vi "Triangle_intersection.vi"(1 "No of Dynamic Facets":i32, 2 "No of Static Facets":i32, 3 "Body Bubble Rad":dbl, 4 "Body Centroid":dbl[](array[numeric]), 5 "Dynamic Facets":T1, 6 "Static Facets":T1) -> (0 "Collision?":bool)   [LabVIEW 2011]
uses:
  Facet_Array.ctl
  <vilib>/Analysis/baseanly.llb/Unit Vector (DBL).vi
  <vilib>/Analysis/baseanly.llb/Real Dot Product.vi
  <vilib>/Analysis/NI_AALBase.lvlib
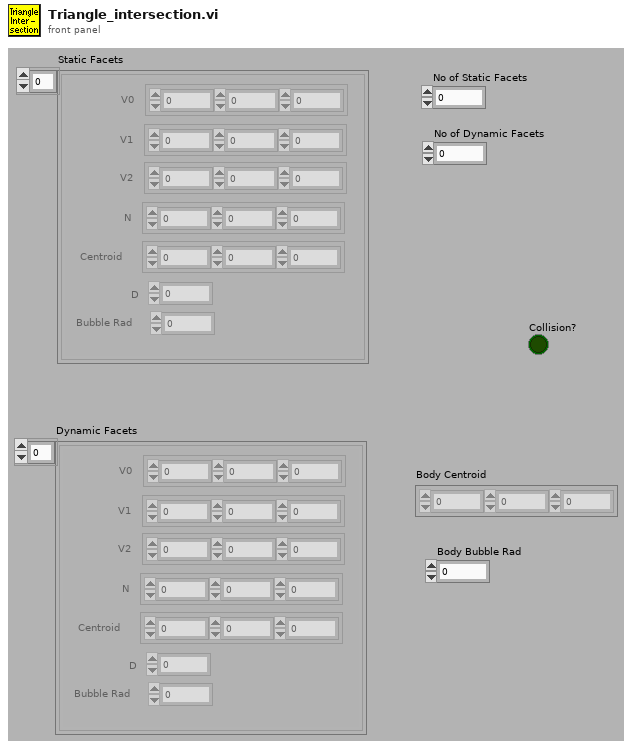
[diagram p1: front panel]
types:
  T1 = typedef "Facet_Array.ctl" = cluster{"V0":dbl[], "V1":dbl[], "V2":dbl[], "N":dbl[], "Centroid":dbl[], "D":dbl, "Bubble Rad":dbl}[]
  T2 = cluster{"V0":dbl[], "V1":dbl[], "V2":dbl[], "N":dbl[], "Centroid":dbl[], "D":dbl, "Bubble Rad":dbl}
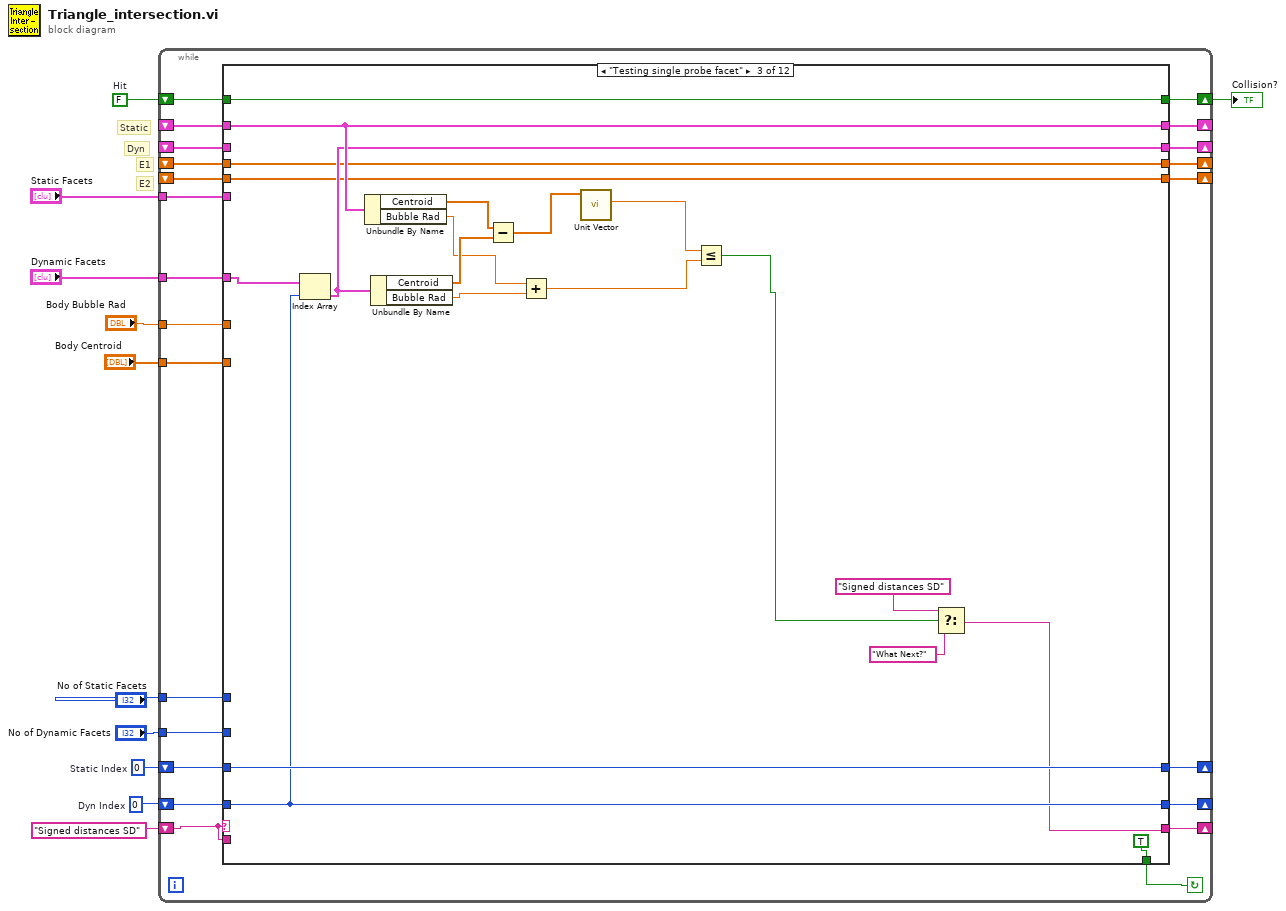
[diagram p0: block diagram]
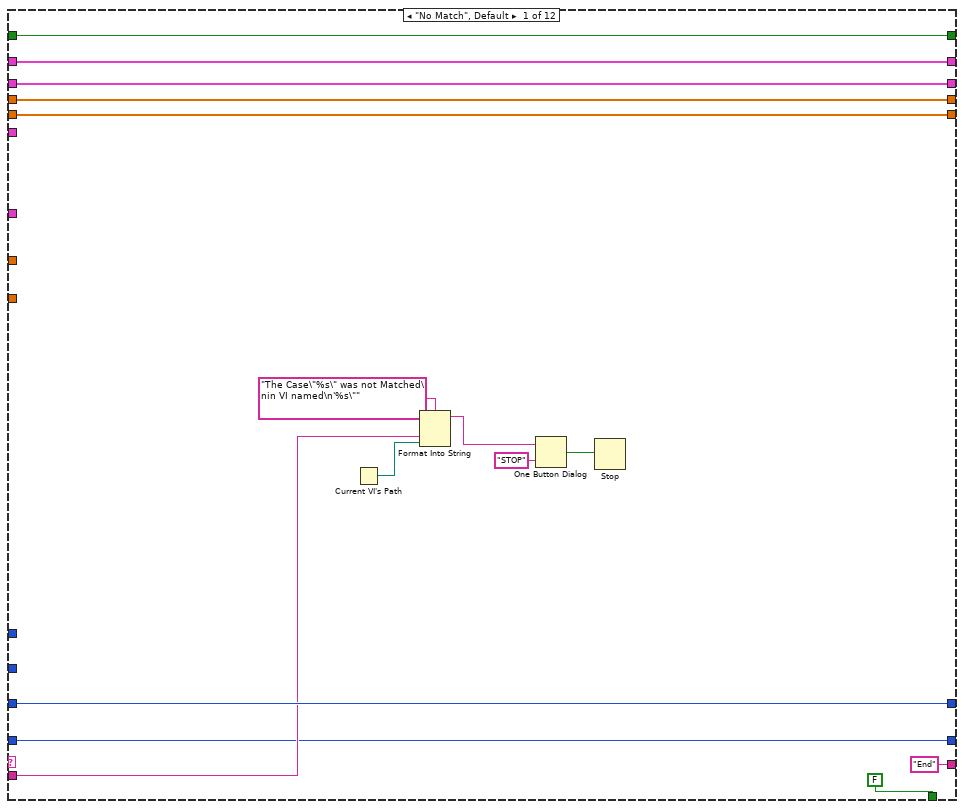
[diagram p2: hidden frame]
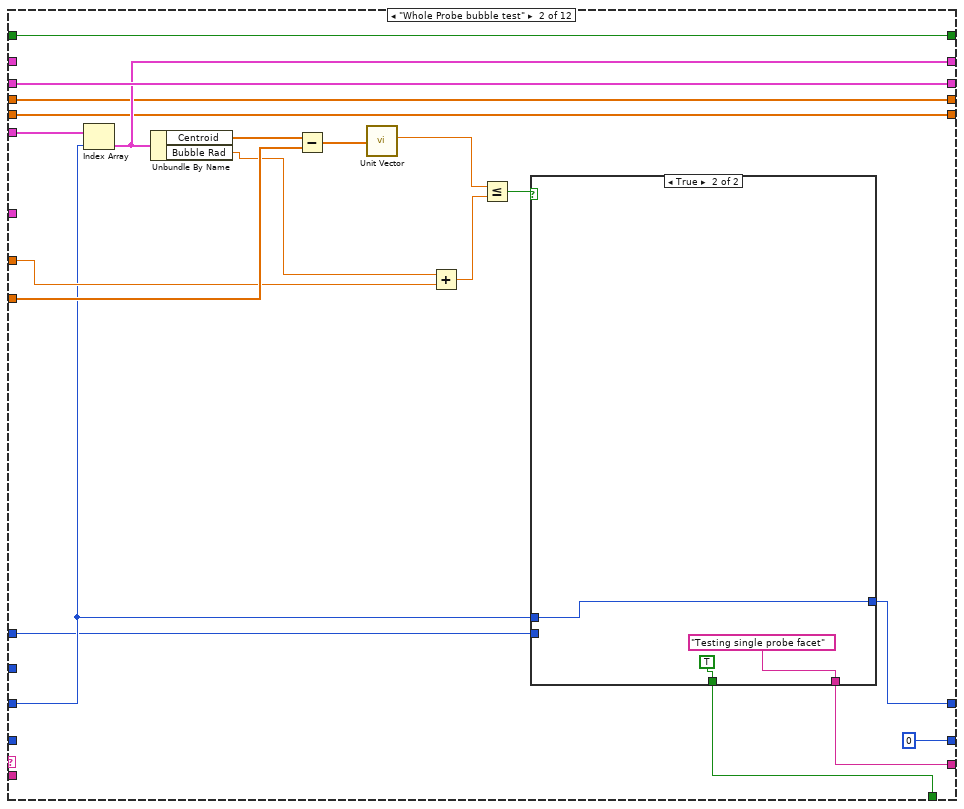
[diagram p3: hidden frame]
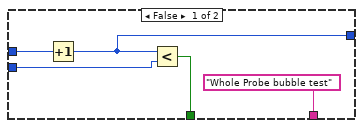
[diagram p4: hidden frame]
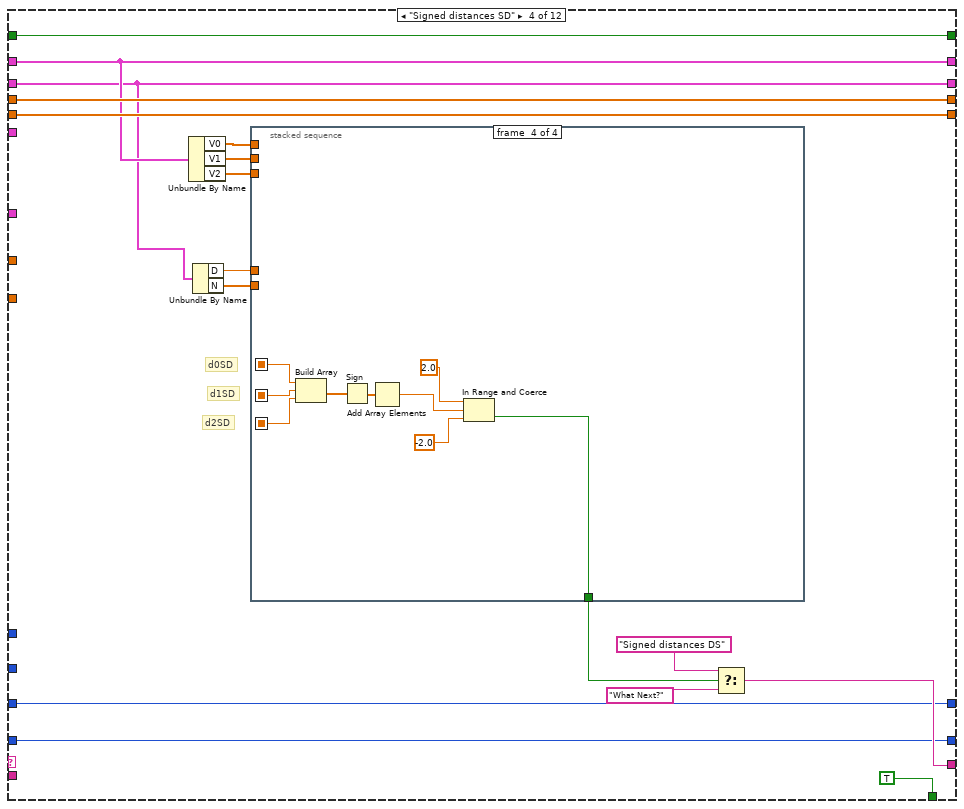
[diagram p5: hidden frame]
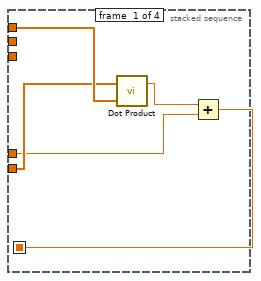
[diagram p6: hidden frame]
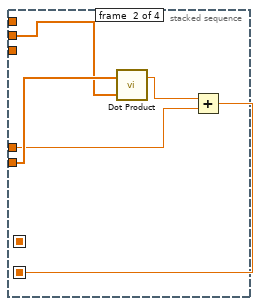
[diagram p7: hidden frame]
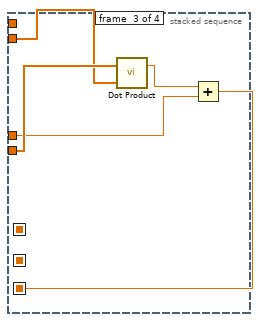
[diagram p8: hidden frame]
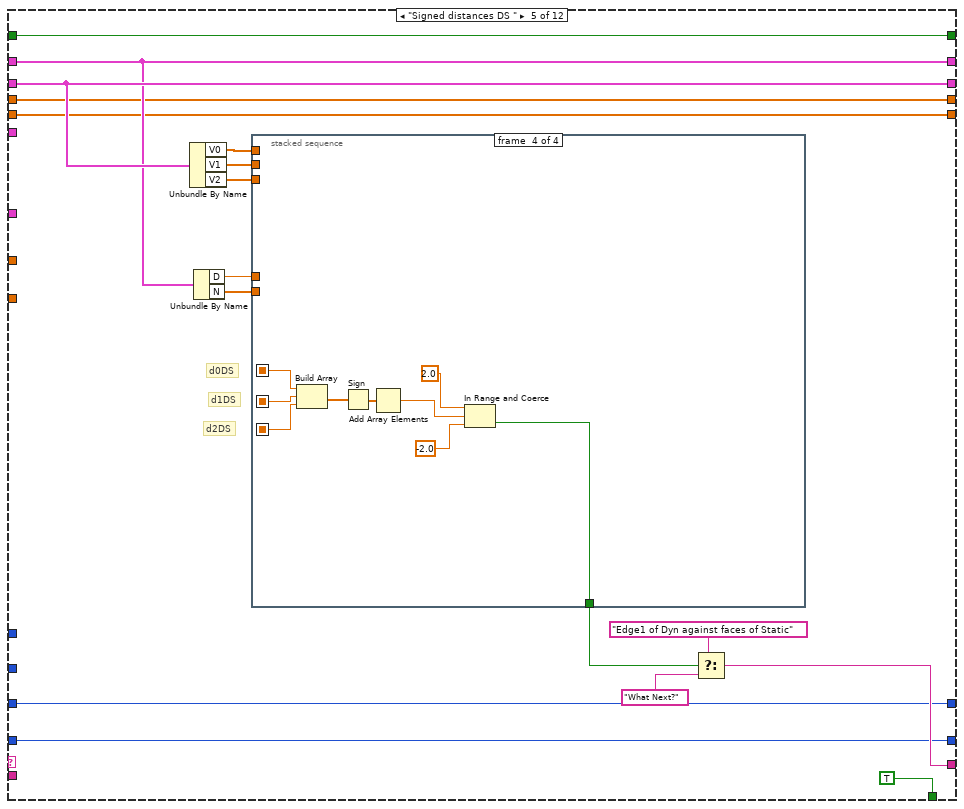
[diagram p9: hidden frame]
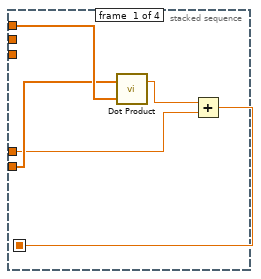
[diagram p10: hidden frame]
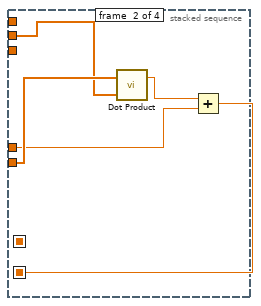
[diagram p11: hidden frame]
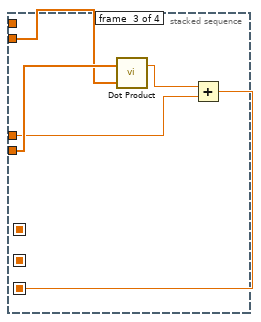
[diagram p12: hidden frame]
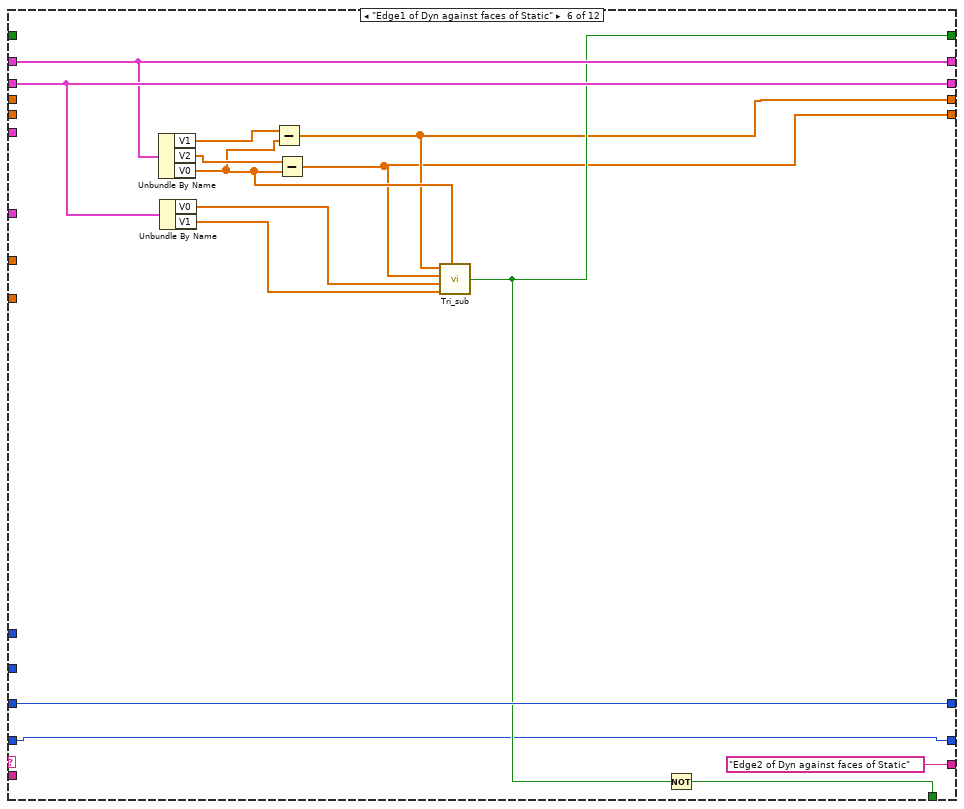
[diagram p13: hidden frame]
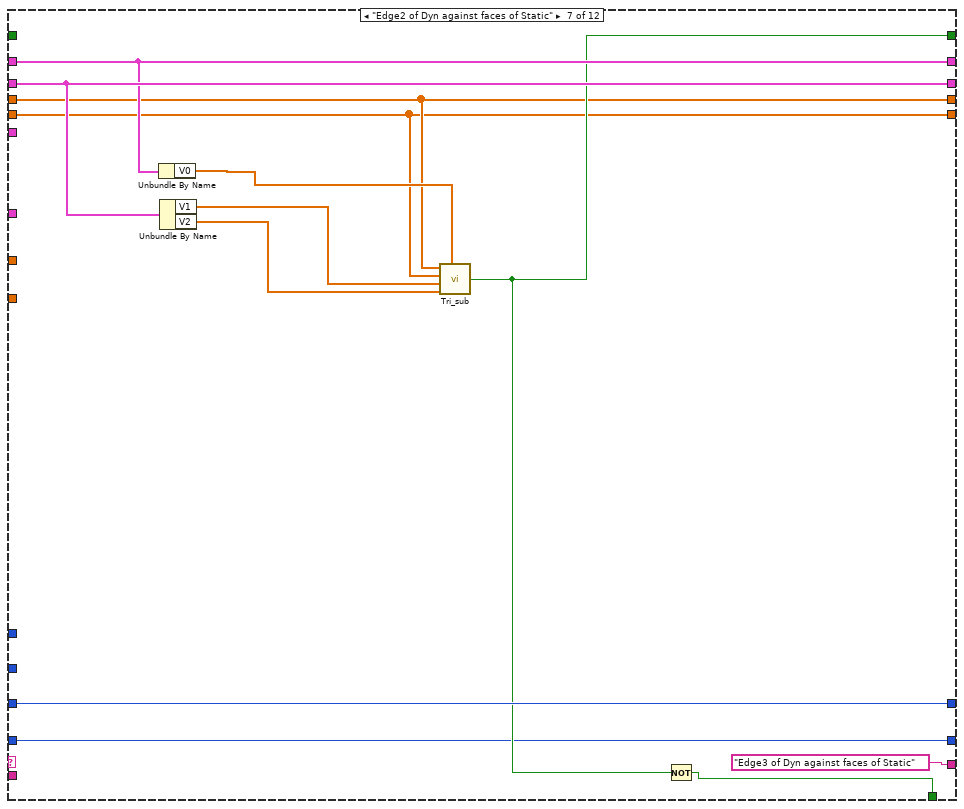
[diagram p14: hidden frame]
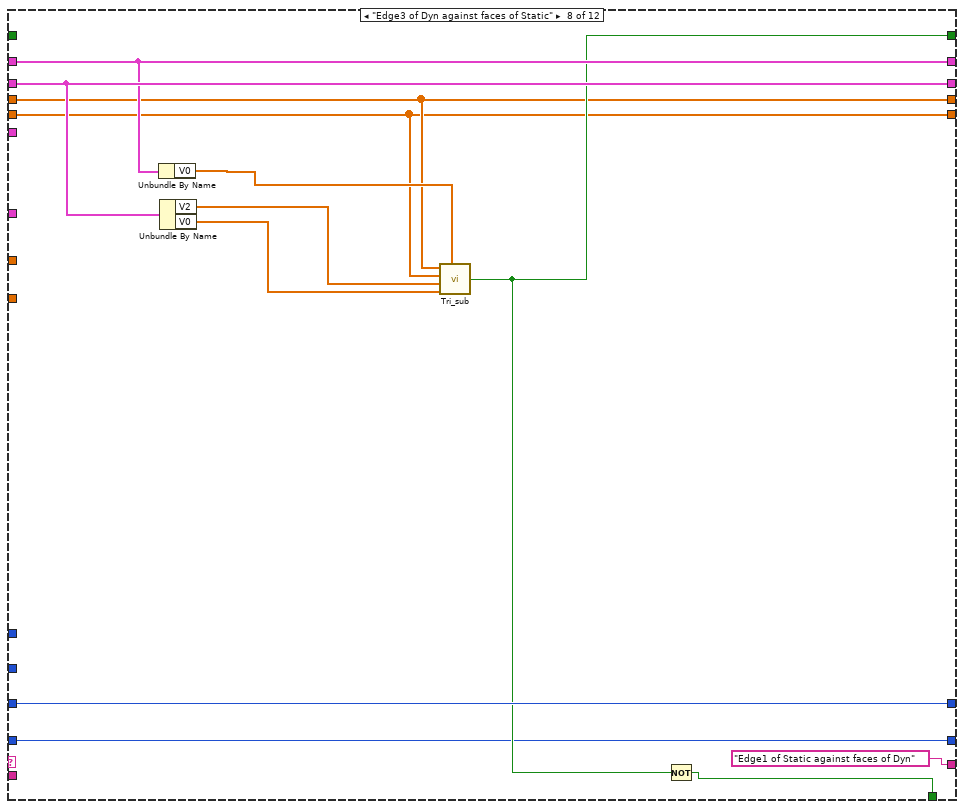
[diagram p15: hidden frame]
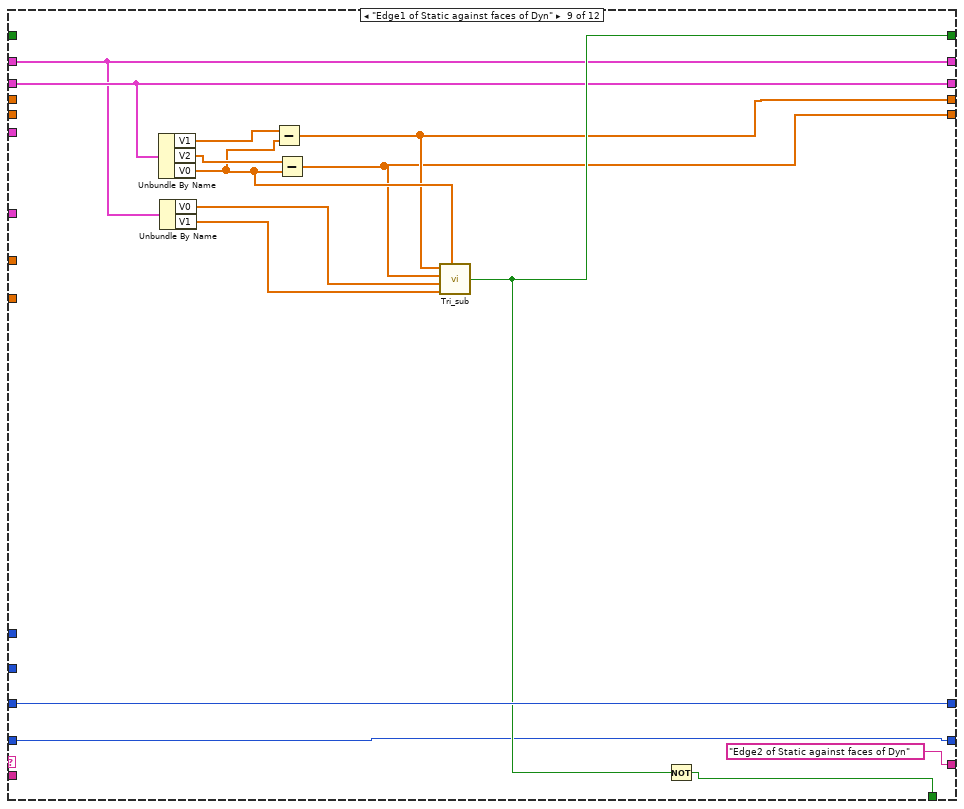
[diagram p16: hidden frame]
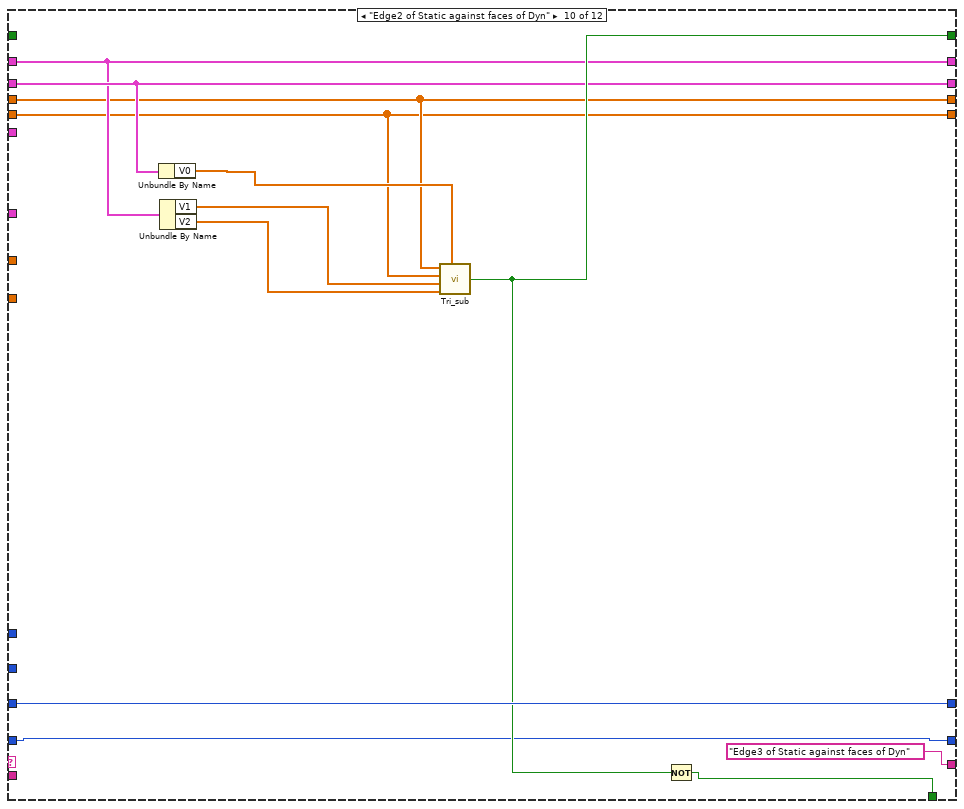
[diagram p17: hidden frame]
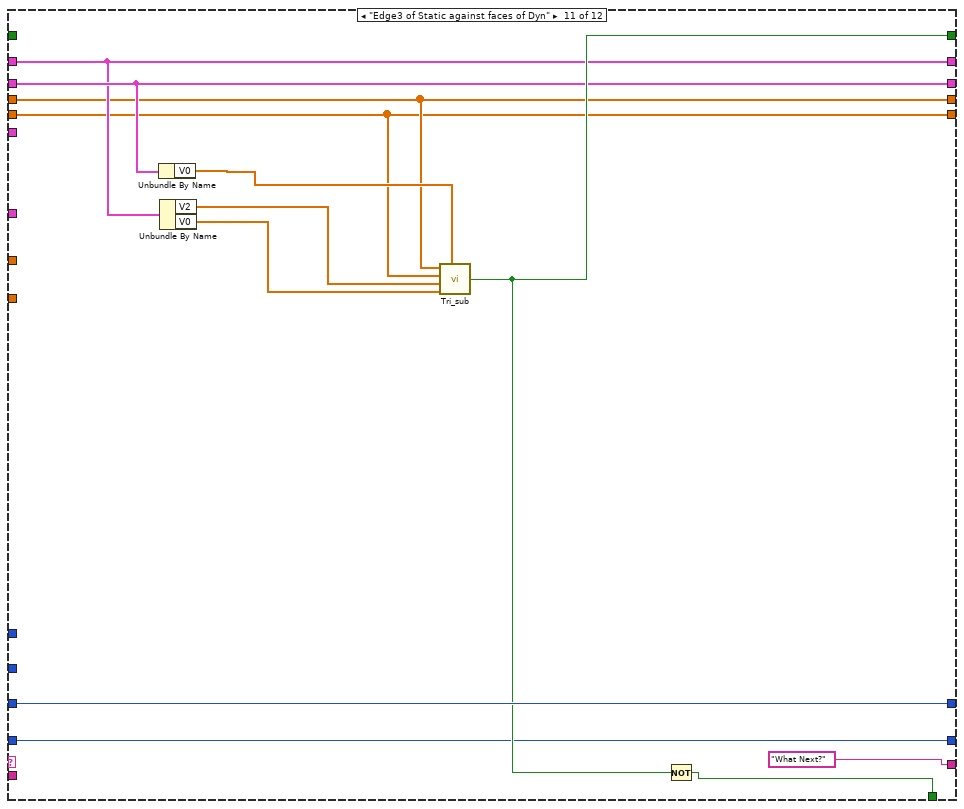
[diagram p18: hidden frame]
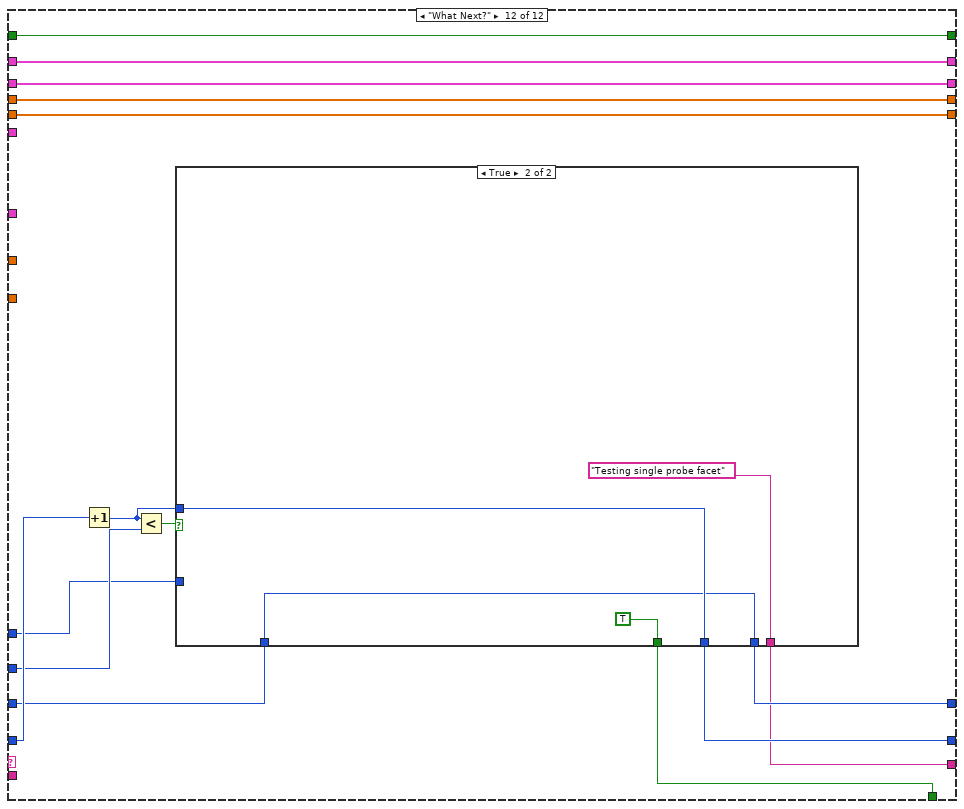
[diagram p19: hidden frame]
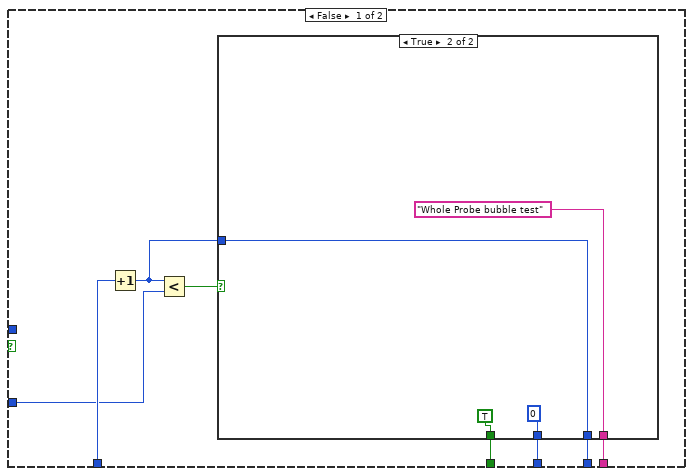
[diagram p20: hidden frame]
diagram:
  w4 = 0  # Dyn Index
  w9 = 0  # Static Index
  w10 = FALSE  # Hit
  # "E2"
  # "E1"
  # "Dyn"
  # "Static"
  n1 = while {
    shift-right: [w28] -> _
    shift-left: "Signed distances SD" -> [w22]
    shift-right: [w26] -> w8
    shift-left: w10 -> [w25]
    shift-right: [w27] -> _
    shift-left: w9 -> [w33]
    tunnel: "Dynamic Facets" -> [w32]
    tunnel: "Static Facets" -> [w31]
    shift-right: [w30] -> _
    shift-left: _ -> [w24]
    shift-right: [w29] -> _
    shift-left: _ -> [w23]
    shift-right: [w21] -> _
    shift-left: _ -> [w19]
    shift-right: [w20] -> _
    shift-left: _ -> [w18]
    tunnel: "Body Centroid" -> [w17]
    tunnel: "Body Bubble Rad" -> [w16]
    shift-right: [w13] -> _
    shift-left: w4 -> [w14]
    tunnel: "No of Static Facets" -> [w15]
    tunnel: "No of Dynamic Facets" -> [w12]
    stop <- w34 continue-if-true
    n2 = case shown="\"Testing single probe facet\"" w22 {
      tunnel: [FALSE w56 TRUE TRUE TRUE w183 w197 w209 w223 w237 w249 w256] -> w34
      tunnel: w33 -> [w46 w58 w86 w104 w145 w193 w205 w217 w231 w243 w255 w259]
      tunnel: w32 -> [_ _ w92 _ _ _ _ _ _ _ _ _]
      tunnel: w31 -> [_ w67 _ _ _ _ _ _ _ _ _ _]
      tunnel: [w48 w65 w93 w100 w142 w191 w203 w215 w219 w235 w247 w269] -> w30
      tunnel: [w47 w68 w91 w99 w143 w192 w204 w216 w220 w236 w248 w268] -> w29
      tunnel: ["End" w55 w78 w105 w146 "Edge2 of Dyn against faces of Static" "Edge3 of Dyn against faces of Static" "Edge1 of Static against faces of Dyn" "Edge2 of Static against faces of Dyn" "Edge3 of Static against faces of Dyn" "What Next?" w257] -> w28
      tunnel: [w46 w54 w86 w104 w145 w193 w205 w217 w231 w243 w255 w260] -> w27
      tunnel: w12 -> [_ _ _ _ _ _ _ _ _ _ _ w264]
      tunnel: [w49 w69 w97 w103 w144 w184 w198 w210 w224 w238 w250 w270] -> w26
      tunnel: w25 -> [w49 w69 w97 w103 w144 _ _ _ _ _ _ w270]
      tunnel: w24 -> [w48 _ w93 w100 w142 w191 w203 w215 w219 w235 w247 w269]
      tunnel: w23 -> [w47 w68 _ w99 w143 w192 w204 w216 w220 w236 w248 w268]
      tunnel: w22 -> [w38 _ _ _ _ _ _ _ _ _ _ _]
      tunnel: [w37 w51 w84 w102 w141 w182 w196 w208 w222 w234 w246 w267] -> w21
      tunnel: [w36 w50 w83 w101 w140 w181 w195 w207 w221 w233 w245 w266] -> w20
      tunnel: w19 -> [w37 w51 w84 w102 w141 _ w196 w208 _ w234 w246 w267]
      tunnel: w18 -> [w36 w50 w83 w101 w140 _ w195 w207 _ w233 w245 w266]
      tunnel: w17 -> [_ w66 _ _ _ _ _ _ _ _ _ _]
      tunnel: w16 -> [_ w60 _ _ _ _ _ _ _ _ _ _]
      tunnel: w15 -> [_ w57 _ _ _ _ _ _ _ _ _ w258]
      tunnel: w14 -> [w35 _ w85 w98 w139 w180 w194 w206 w218 w232 w244 w265]
      tunnel: [w35 0 w85 w98 w139 w180 w194 w206 w218 w232 w244 w262] -> w13
      frame "No Match", Default {
        n3 = Current VI's Path() -> (path=w43:path)
        n4 = Format Into String(format string="The Case\"%s\" was not Matched\nin VI named\n'%s\"" ("Format String"), w38, w43) -> (resulting string=w40:string)  [unwired: 2 in, 1 out]
        n5 = One Button Dialog(message=w40, button name ("OK")="STOP") -> (true=w42:bool)
        n6 = Stop(stop? (T)=w42) -> ()
      }
      frame "Whole Probe bubble test" {
        n7 = Index Array(array=w67, index=w58) -> (element=w65:T2)
        n8 = Unbundle By Name(w65) -> ("Centroid"=w52:dbl[], "Bubble Rad"=w61:dbl)
        n9 = Subtract(x=w52, y=w66) -> (x-y=w64:dbl[])
        n10 = call-poly <vilib>:"Unit Vector.vi"("Input Vector"=w64) -> ("norm"=w63:dbl)  [unwired: 2 in, 8 out]
        n11 = Add(x=w61, y=w60) -> (x+y=w62:dbl)
        n12 = Less Or Equal?(x=w63, y=w62) -> (x <= y?=w59:bool)
        n13 = case shown="True" w59 {
          tunnel: w58 -> [w74 w75]
          tunnel: w57 -> [w73 _]
          tunnel: [w72 TRUE] -> w56
          tunnel: ["Whole Probe bubble test" "Testing single probe facet"] -> w55
          tunnel: [w70 w75] -> w54
          frame False {
            n14 = Increment(x=w74) -> (x+1=w70:i32)
            n15 = Less?(x=w70, y=w73) -> (x < y?=w72:bool)
          }
          frame True {
          }
        }
      }
      frame "Testing single probe facet" {
        n16 = Index Array(array=w92, index=w85) -> (element=w91:T2)
        n17 = Unbundle By Name(w93) -> ("Centroid"=w89:dbl[], "Bubble Rad"=w87:dbl)
        n18 = Unbundle By Name(w91) -> ("Centroid"=w90:dbl[], "Bubble Rad"=w88:dbl)
        n19 = Subtract(x=w89, y=w90) -> (x-y=w96:dbl[])
        n20 = Add(x=w87, y=w88) -> (x+y=w94:dbl)
        n21 = call-poly <vilib>:"Unit Vector.vi"("Input Vector"=w96) -> ("norm"=w95:dbl)  [unwired: 2 in, 8 out]
        n22 = Less Or Equal?(x=w95, y=w94) -> (x <= y?=w79:bool)
        n23 = Select(t="Signed distances SD", s=w79, f="What Next?") -> (s? t:f=w78:string)
      }
      frame "Signed distances SD" {
        # "d2SD"
        # "d1SD"
        # "d0SD"
        n24 = Unbundle By Name(w100) -> ("V0"=w113:dbl[], "V1"=w110:dbl[], "V2"=w109:dbl[])
        n25 = Unbundle By Name(w99) -> ("D"=w111:dbl, "N"=w112:dbl[])
        n26 = stacked-sequence {
          seq-local: [w118 _ _ _] -> [_ _ _ w138]
          seq-local: [_ w121 _ _] -> [_ _ _ w137]
          seq-local: [_ _ w126 _] -> [_ _ _ w136]
          tunnel: w113 -> [w117 _ _ _]
          tunnel: w112 -> [w116 w123 w128 _]
          tunnel: w111 -> [w115 w122 w127 _]
          tunnel: w110 -> [_ w120 _ _]
          tunnel: w109 -> [_ _ w125 _]
          tunnel: [_ _ _ w130] -> w108
          frame #0 {
            n27 = call-poly <vilib>:"Dot Product.vi"("Y Vector"=w117, "X Vector"=w116) -> ("X * Y"=w119:dbl)  [unwired: 1 out]
            n28 = Add(x=w119, y=w115) -> (x+y=w118:dbl)
          }
          frame #1 {
            n29 = call-poly <vilib>:"Dot Product.vi"("Y Vector"=w120, "X Vector"=w123) -> ("X * Y"=w124:dbl)  [unwired: 1 out]
            n30 = Add(x=w124, y=w122) -> (x+y=w121:dbl)
          }
          frame #2 {
            n31 = call-poly <vilib>:"Dot Product.vi"("Y Vector"=w125, "X Vector"=w128) -> ("X * Y"=w129:dbl)  [unwired: 1 out]
            n32 = Add(x=w129, y=w127) -> (x+y=w126:dbl)
          }
          frame #3 {
            n33 = Build Array(w138, w137, w136) -> (w135:dbl[])
            n34 = Sign(1:w135) -> (0:w134:dbl[])
            n35 = Add Array Elements(numeric array=w134) -> (sum=w133:dbl)
            n36 = In Range and Coerce(upper limit=2.0, x=w133, lower limit=-2.0) -> (In Range?=w130:bool)  [unwired: 1 out]
          }
        }
        n37 = Select(t="Signed distances DS", s=w108, f="What Next?") -> (s? t:f=w105:string)
      }
      frame "Signed distances DS " {
        # "d2DS"
        # "d1DS"
        # "d0DS"
        n38 = Unbundle By Name(w143) -> ("V0"=w154:dbl[], "V1"=w151:dbl[], "V2"=w150:dbl[])
        n39 = Unbundle By Name(w142) -> ("D"=w152:dbl, "N"=w153:dbl[])
        n40 = stacked-sequence {
          seq-local: [w159 _ _ _] -> [_ _ _ w179]
          seq-local: [_ w162 _ _] -> [_ _ _ w178]
          seq-local: [_ _ w167 _] -> [_ _ _ w177]
          tunnel: w154 -> [w158 _ _ _]
          tunnel: w153 -> [w157 w164 w169 _]
          tunnel: w152 -> [w156 w163 w168 _]
          tunnel: w151 -> [_ w161 _ _]
          tunnel: w150 -> [_ _ w166 _]
          tunnel: [_ _ _ w171] -> w149
          frame #0 {
            n41 = call-poly <vilib>:"Dot Product.vi"("Y Vector"=w158, "X Vector"=w157) -> ("X * Y"=w160:dbl)  [unwired: 1 out]
            n42 = Add(x=w160, y=w156) -> (x+y=w159:dbl)
          }
          frame #1 {
            n43 = call-poly <vilib>:"Dot Product.vi"("Y Vector"=w161, "X Vector"=w164) -> ("X * Y"=w165:dbl)  [unwired: 1 out]
            n44 = Add(x=w165, y=w163) -> (x+y=w162:dbl)
          }
          frame #2 {
            n45 = call-poly <vilib>:"Dot Product.vi"("Y Vector"=w166, "X Vector"=w169) -> ("X * Y"=w170:dbl)  [unwired: 1 out]
            n46 = Add(x=w170, y=w168) -> (x+y=w167:dbl)
          }
          frame #3 {
            n47 = Build Array(w179, w178, w177) -> (w176:dbl[])
            n48 = Sign(1:w176) -> (0:w175:dbl[])
            n49 = Add Array Elements(numeric array=w175) -> (sum=w174:dbl)
            n50 = In Range and Coerce(upper limit=2.0, x=w174, lower limit=-2.0) -> (In Range?=w171:bool)  [unwired: 1 out]
          }
        }
        n51 = Select(t="Edge1 of Dyn against faces of Static", s=w149, f="What Next?") -> (s? t:f=w146:string)
      }
      frame "Edge1 of Dyn against faces of Static" {
        n52 = Unbundle By Name(w191) -> ("V1"=w190:dbl[], "V2"=w189:dbl[], "V0"=w186:dbl[])
        n53 = Unbundle By Name(w192) -> ("V0"=w188:dbl[], "V1"=w187:dbl[])
        n54 = Subtract(x=w190, y=w186) -> (x-y=w182:dbl[])
        n55 = Subtract(x=w189, y=w186) -> (x-y=w181:dbl[])
        n56 = call "Tri_sub.vi"("E1"=w182, "E2"=w181, "O0"=w188, "O1"=w187, "V0"=w186) -> ("Collision?"=w184:bool)
        n57 = Not(x=w184) -> (.not. x?=w183:bool)
      }
      frame "Edge2 of Dyn against faces of Static" {
        n58 = Unbundle By Name(w203) -> ("V0"=w200:dbl[])
        n59 = Unbundle By Name(w204) -> ("V1"=w202:dbl[], "V2"=w201:dbl[])
        n60 = call "Tri_sub.vi"("E1"=w196, "E2"=w195, "O0"=w202, "O1"=w201, "V0"=w200) -> ("Collision?"=w198:bool)
        n61 = Not(x=w198) -> (.not. x?=w197:bool)
      }
      frame "Edge3 of Dyn against faces of Static" {
        n62 = Unbundle By Name(w215) -> ("V0"=w212:dbl[])
        n63 = Unbundle By Name(w216) -> ("V2"=w214:dbl[], "V0"=w213:dbl[])
        n64 = call "Tri_sub.vi"("E1"=w208, "E2"=w207, "O0"=w214, "O1"=w213, "V0"=w212) -> ("Collision?"=w210:bool)
        n65 = Not(x=w210) -> (.not. x?=w209:bool)
      }
      frame "Edge1 of Static against faces of Dyn" {
        n66 = Unbundle By Name(w220) -> ("V1"=w230:dbl[], "V2"=w229:dbl[], "V0"=w226:dbl[])
        n67 = Unbundle By Name(w219) -> ("V0"=w228:dbl[], "V1"=w227:dbl[])
        n68 = Subtract(x=w230, y=w226) -> (x-y=w222:dbl[])
        n69 = Subtract(x=w229, y=w226) -> (x-y=w221:dbl[])
        n70 = call "Tri_sub.vi"("E1"=w222, "E2"=w221, "O0"=w228, "O1"=w227, "V0"=w226) -> ("Collision?"=w224:bool)
        n71 = Not(x=w224) -> (.not. x?=w223:bool)
      }
      frame "Edge2 of Static against faces of Dyn" {
        n72 = Unbundle By Name(w236) -> ("V0"=w240:dbl[])
        n73 = Unbundle By Name(w235) -> ("V1"=w242:dbl[], "V2"=w241:dbl[])
        n74 = call "Tri_sub.vi"("E1"=w234, "E2"=w233, "O0"=w242, "O1"=w241, "V0"=w240) -> ("Collision?"=w238:bool)
        n75 = Not(x=w238) -> (.not. x?=w237:bool)
      }
      frame "Edge3 of Static against faces of Dyn" {
        n76 = Unbundle By Name(w248) -> ("V0"=w252:dbl[])
        n77 = Unbundle By Name(w247) -> ("V2"=w254:dbl[], "V0"=w253:dbl[])
        n78 = call "Tri_sub.vi"("E1"=w246, "E2"=w245, "O0"=w254, "O1"=w253, "V0"=w252) -> ("Collision?"=w250:bool)
        n79 = Not(x=w250) -> (.not. x?=w249:bool)
      }
      frame "What Next?" {
        n80 = Increment(x=w265) -> (x+1=w261:i32)
        n81 = Less?(x=w261, y=w264) -> (x < y?=w263:bool)
        n82 = case shown="True" w263 {
          tunnel: [w273 w290] -> w262
          tunnel: w261 -> [_ w290]
          tunnel: [w274 w289] -> w260
          tunnel: w259 -> [w278 w289]
          tunnel: w258 -> [w277 _]
          tunnel: [w272 "Testing single probe facet"] -> w257
          tunnel: [w271 TRUE] -> w256
          frame False {
            n83 = Increment(x=w278) -> (x+1=w275:i32)
            n84 = Less?(x=w275, y=w277) -> (x < y?=w276:bool)
            n85 = case shown="True" w276 {
              tunnel: w275 -> [_ w286]
              tunnel: [0 w286] -> w274
              tunnel: [0 0] -> w273
              tunnel: ["End" "Whole Probe bubble test"] -> w272
              tunnel: [FALSE TRUE] -> w271
              frame False {
              }
              frame True {
              }
            }
          }
          frame True {
          }
        }
      }
    }
  }
  "Collision?" <- w8
